vi "{{Message}}.vi"(6 "Error":errorcluster, 7 "Actor":refnum<class "Actor.lvclass">, 11 "Message":refnum<class "Message.lvclass">) -> (3 "Message":refnum<class "Message.lvclass">, 4 "Error":errorcluster, 5 "Actor":refnum<class "Actor.lvclass">)   [LabVIEW 2020, in "_Template.lvlib" / "{{Actor}}.lvlib" / "Actor.lvclass"]
uses:
  Actor.lvclass
  C:/jettl-harness/repos/jettl/src/jettl/jettl/Actor/Actor.lvclass
  {{Message}}/Message/Message.lvclass
  C:/jettl-harness/repos/jettl/src/jettl/jettl/Message/Message.lvclass
  jettl/jettl/Actor/Actor.lvclass
  {{Message}}/{{Message}}.lvlib
panel:
  # "This front panel should not be manipulated."
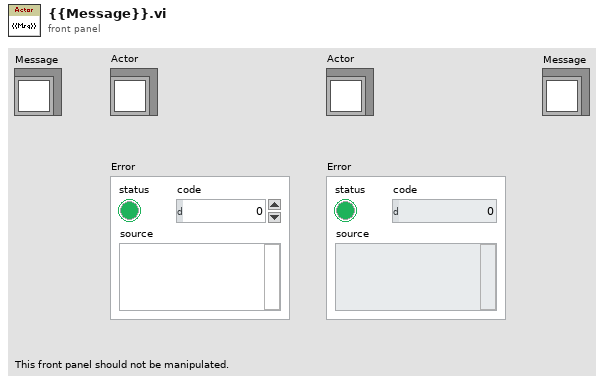
[diagram p1: front panel]
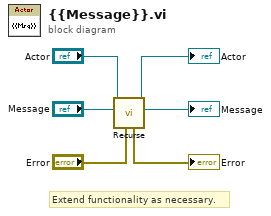
[diagram p0: block diagram]
diagram:
  # "Extend functionality as necessary."
  n1 = call "Recurse.vi"("Error"="Error", "Message"="Message", "Actor"="Actor") -> ("Message"=→"Message":refnum<class "Message.lvclass">, "Actor"=→"Actor":refnum<class "Actor.lvclass">, "Error"=→"Error":errorcluster)  [unwired: 6 in]
